vi "OrExpression.vi"(8 "error in (no error)":errorcluster, 9 "expr2":refnum<class "TerminalExpression.lvclass">, 10 "expr1":refnum<class "TerminalExpression.lvclass">, 11 "OrExpression in":refnum<class "OrExpression.lvclass">) -> (0 "error out":errorcluster, 3 "OrExpression out":refnum<class "OrExpression.lvclass">)   [LabVIEW 2018, in "OrExpression.lvclass"]
uses:
  OrExpression.lvclass
  TerminalExpression Class/TerminalExpression.lvclass
  OrExpression.lvclass/OrExpression.ctl
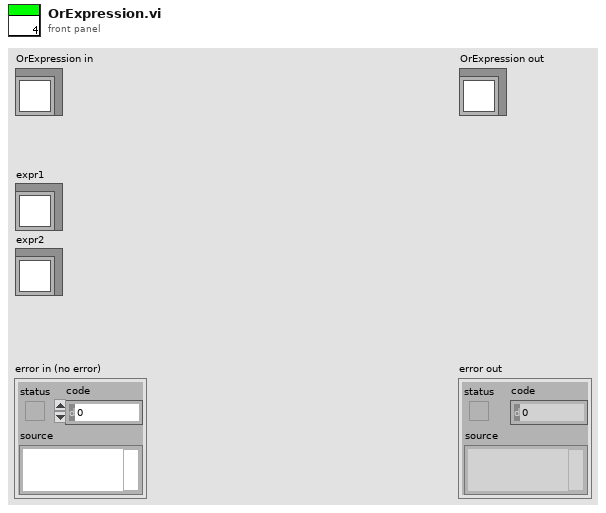
[diagram p1: front panel]
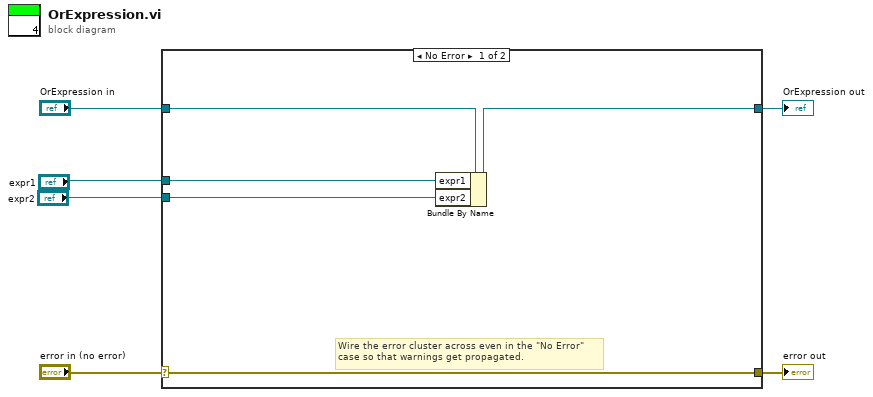
[diagram p0: block diagram]
diagram:
  n1 = case shown="No Error" "error in (no error)" {
    selector: "error in (no error)" -> [w10 w13]
    tunnel: [w10 w13] -> w5
    tunnel: [w9 w12] -> w3
    tunnel: "OrExpression in" -> [w11 w12]
    tunnel: "expr1" -> [w8 _]
    tunnel: "expr2" -> [w7 _]
    frame No Error {
      # "Wire the error cluster across even in the \"No Error\"\ncase so that warnings get propagated."
      n2 = Bundle By Name(cluster=w11, "expr1"=w8, "expr2"=w7) -> (w9:refnum<class "OrExpression.lvclass">)
    }
    frame Error {
    }
  }
  "error out" <- w5
  "OrExpression out" <- w3
